vi "CallDestructor.vi"(10 "ActorLightIn":refnum<class "YActor.lvclass">, 11 "Array":string[](array[string])) -> (3 "YActorOut":refnum<class>)   [LabVIEW 2021, in "YActor.lvclass"]
doc: "Called at the destruction of the object. Use this to clear references or perform action to tidy up the object."
uses:
  YActor.lvclass
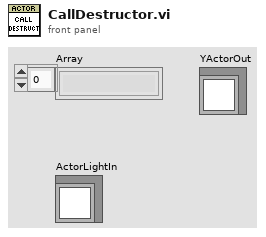
[diagram p1: front panel]
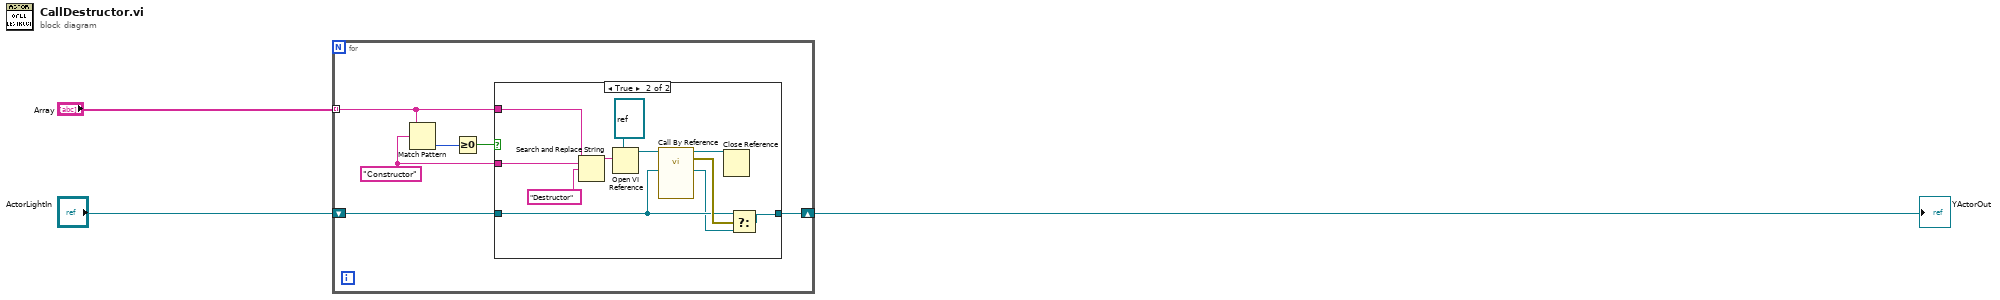
[diagram p0: block diagram]
diagram:
  n1 = for {
    shift-right: [w7] -> w1
    shift-left: "ActorLightIn" -> [w8]
    tunnel: "Array" -> [w4] mode=indexing
    w5 = "Constructor" ("search string")
    n2 = Match Pattern(string=w4, regular expression=w5) -> (offset past match=w9:i32)  [unwired: 1 in, 3 out]
    n3 = Greater Or Equal To 0?(x=w9) -> (x >= 0?=w6:bool)
    n4 = case shown="True" w6 {
      tunnel: w8 -> [w10 w15]
      tunnel: [w10 w13] -> w7
      tunnel: w5 -> [_ w12]
      tunnel: w4 -> [_ w11]
      frame False {
      }
      frame True {
        n5 = Search and Replace String(input string=w11, search string=w12, replace string="Destructor" ("replace string (\"\")")) -> (result string=w18:string)  [unwired: 5 in, 3 out]
        n6 = Open VI Reference(type specifier VI Refnum (for type only)=refnum<vi> refnum, vi path=w18) -> (vi reference=w17:refnum<vi>)  [unwired: 4 in, 1 out]
        n7 = call-by-ref "?"(reference=w17, "Local in"=w15) -> (reference out=w16:refnum<vi>, error out=w21:errorcluster, "Local out"=w14:refnum<class>)  [unwired: 8 in, 3 out]
        n8 = Close Reference(reference=w16) -> ()  [unwired: 1 in, 1 out]
        n9 = Select(t=w15, s=w21, f=w14) -> (s? t:f=w13:refnum<class>)
      }
    }
  }
  "YActorOut" <- w1
